vi "Build Tasks.vi"(7 "TaskName":string, 8 "error in (no error)":errorcluster, 9 "writeCh":tag[](array[tag]), 10 "readCh":tag[](array[tag]), 11 "DAQmxSwitch in":refnum<class "DAQmxSwitch.lvclass">) -> (0 "error out":errorcluster, 3 "DAQmxSwitch out":refnum<class "DAQmxSwitch.lvclass">)   [LabVIEW 2009, in "DAQmxSwitch.lvclass"]
uses:
  DAQmxSwitch.lvclass
  <vilib>/DAQmx/create/channels.llb/DAQmx Create Channel (DI-Digital Input).vi
  <vilib>/DAQmx/create/channels.llb/DAQmx Create Channel (DO-Digital Output).vi
  DAQmxSwitch.lvclass/DAQmxSwitch.ctl
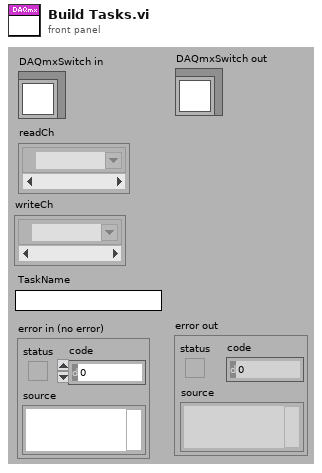
[diagram p1: front panel]
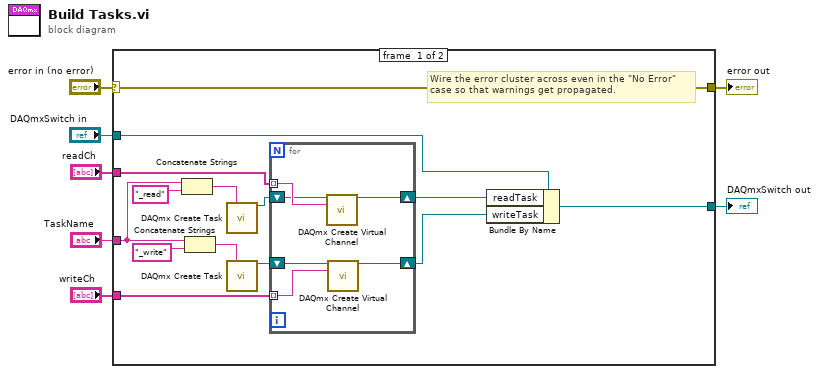
[diagram p0: block diagram]
diagram:
  n1 = case shown="No Error" "error in (no error)" {
    selector: "error in (no error)" -> [w21 w29]
    tunnel: [w21 w29] -> w6
    tunnel: [w8 w28] -> w4
    tunnel: "DAQmxSwitch in" -> [w11 w28]
    tunnel: "readCh" -> [w20 _]
    tunnel: "TaskName" -> [w15 _]
    tunnel: "writeCh" -> [w16 _]
    frame #0 {
      # "Wire the error cluster across even in the \"No Error\"\ncase so that warnings get propagated."
      n2 = Concatenate Strings(w15, "_read" ("string")) -> (w18:string)
      n3 = Concatenate Strings(w15, "_write" ("string")) -> (w13:string)
      n4 = call <vilib>:"DAQmx Create Task.vi"("new task name"=w18) -> ("task out"=w17:refnum<k21>)  [unwired: 13 in, 1 out]
      n5 = call <vilib>:"DAQmx Create Task.vi"("new task name"=w13) -> ("task out"=w12:refnum<k21>)  [unwired: 13 in, 1 out]
      n6 = for {
        tunnel: w20 -> [w27] mode=indexing
        shift-right: [w25] -> w10
        shift-left: w17 -> [w26]
        tunnel: w16 -> [w24] mode=indexing
        shift-right: [w23] -> w9
        shift-left: w12 -> [w22]
        n7 = call-poly <vilib>:"DAQmx Create Virtual Channel.vi"("task in"=w26, "lines"=w27) -> ("task out"=w25:refnum<k21>)  [unwired: 12 in, 1 out]
        n8 = call-poly <vilib>:"DAQmx Create Virtual Channel.vi"("task in"=w22, "lines"=w24) -> ("task out"=w23:refnum<k21>)  [unwired: 12 in, 1 out]
      }
      n9 = Bundle By Name(cluster=w11, "readTask"=w10, "writeTask"=w9) -> (w8:refnum<class "DAQmxSwitch.lvclass">)
    }
    frame #1 {
    }
  }
  "error out" <- w6
  "DAQmxSwitch out" <- w4
